vi "Open Shutter.vi"(8 "error in (no error)":errorcluster, 9 "ALEX?":bool, 10 "Selected lasers":bool[](array[boolean])=[FALSE, FALSE, FALSE, FALSE], 11 "Synchronization Device in":refnum<class "Microsync.lvclass">) -> (0 "error out":errorcluster, 3 "Synchronization Device out":refnum<class "Microsync.lvclass">)   [LabVIEW 2023, in "Microsync.lvlib" / "Microsync.lvclass"]
uses:
  Microsync.lvclass
  Microsync.lvclass/Microsync.ctl
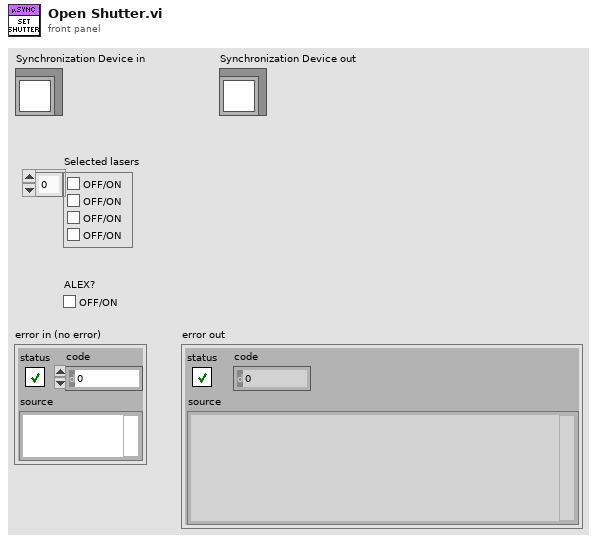
[diagram p1: front panel]
types:
  T1 = enum16{"ro_VERSION", "ro_SYS_TIMER_STATUS", "ro_SYS_TIMER_VALUE", "ro_SYS_TIMER_OVF_COUNT", "ro_SYS_TIME_ms", "ro_SYS_TIMER_PRESCALER", "rw_DFLT_PULSE_DURATION_us", "ro_WATCHDOG_TIMEOUT_ms", "ro_N_EVENTS", "rw_INTLCK_ENABLED", "rw_SELECTED_LASERS", "wo_OPEN_SHUTTERS", "wo_CLOSE_SHUTTERS", "rw_SHUTTER_DELAY_us", "rw_CAM_READOUT_us"}
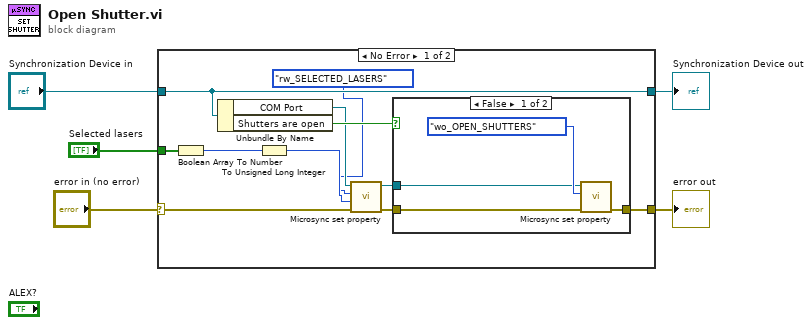
[diagram p0: block diagram]
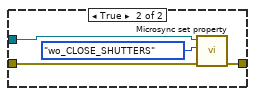
[diagram p2: hidden frame]
diagram:
  n1 = case shown="No Error" "error in (no error)" {
    selector: "error in (no error)" -> [w8 w25]
    tunnel: "Synchronization Device in" -> [w14 w26]
    tunnel: "Selected lasers" -> [w15 _]
    tunnel: [w10 w25] -> w2
    tunnel: [w14 w26] -> w1
    frame No Error {
      n2 = Boolean Array To Number(Boolean array=w15) -> (number=w16:u32)
      n3 = Unbundle By Name(w14) -> ("COM Port"=w9:refnum<visa-resource-name>, "Shutters are open"=w13:bool)
      n4 = To Unsigned Long Integer(number=w16) -> (unsigned 32bit integer=w7:u32)
      n5 = call "Microsync set property.vi"("error in (no error)"=w8, "Property value"=w7, "property to set"=T1."rw_SELECTED_LASERS" ("property"), "VISA resource name"=w9) -> ("error out"=w12:errorcluster, "VISA resource name out"=w11:refnum<visa-resource-name>)  [unwired: 6 in]
      n6 = case shown="False" w13 {
        tunnel: w12 -> [w18 w21]
        tunnel: w11 -> [w17 w23]
        tunnel: [w20 w24] -> w10
        frame False {
          n7 = call "Microsync set property.vi"("error in (no error)"=w18, "property to set"=T1."wo_OPEN_SHUTTERS" ("property"), "VISA resource name"=w17) -> ("error out"=w20:errorcluster)  [unwired: 7 in, 1 out]
        }
        frame True {
          n8 = call "Microsync set property.vi"("error in (no error)"=w21, "property to set"=T1."wo_CLOSE_SHUTTERS" ("property"), "VISA resource name"=w23) -> ("error out"=w24:errorcluster)  [unwired: 7 in, 1 out]
        }
      }
    }
    frame Error {
    }
  }
  "error out" <- w2
  "Synchronization Device out" <- w1
